vi "Fit.vi"(7 "Type X":T1(ring), 8 "error in (no error)":errorcluster caption="entrée d'erreur (pas d'erreur)", 9 "y":string[][](array[string]), 10 "X":string[][](array[string]), 11 "GaussianRandomProjection.lvclass":refnum<class "GaussianRandomProjection.lvclass">) -> (0 "error out":errorcluster caption="sortie d'erreur", 2 "String Data":string, 3 "GaussianRandomProjection.lvclass":refnum<class "GaussianRandomProjection.lvclass">)   [LabVIEW 2020, in "GaussianRandomProjection.lvclass"]
doc: "Generate a sparse random projection matrix\n\nReturns : \n\n- String : OK"
uses:
  GaussianRandomProjection.lvclass
  GaussianRandomProjection.lvclass/GaussianRandomProjection.ctl
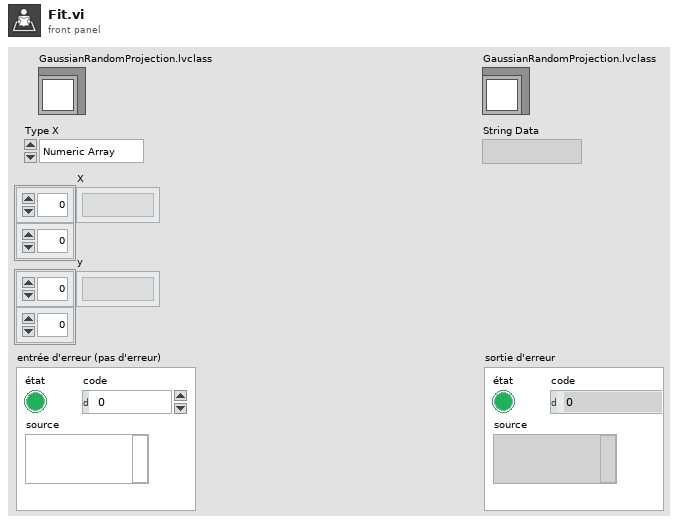
[diagram p1: front panel]
types:
  T1 = enum16{"Numeric Array", "String Array", "Sparse"}
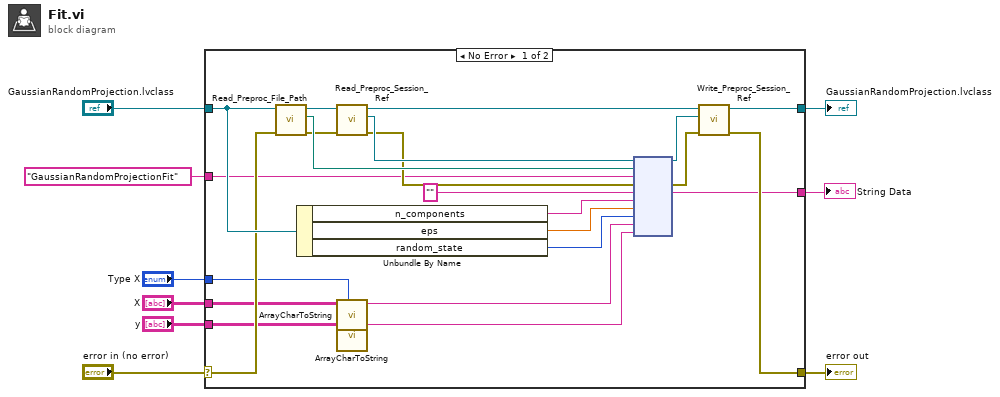
[diagram p0: block diagram]
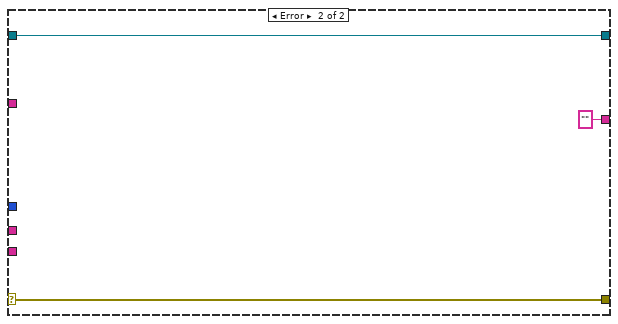
[diagram p2: hidden frame]
diagram:
  n1 = case shown="No Error" "error in (no error)" {
    selector: "error in (no error)" -> [w21 w35]
    tunnel: [w20 w35] -> w8
    tunnel: [w22 w34] -> w6
    tunnel: "GaussianRandomProjection.lvclass" -> [w23 w34]
    tunnel: "GaussianRandomProjectionFit" ("Fonction") -> [w19 _]
    tunnel: [w18 ""] -> w4
    tunnel: "X" -> [w14 _]
    tunnel: "y" -> [w13 _]
    tunnel: "Type X" -> [w12 _]
    frame No Error {
      n2 = call-dynamic "Read_Preproc_File_Path.vi"("error in (no error)"=w21, "Python in"=w23) -> ("error out"=w27:errorcluster, "File_Path"=w30:path, "Python out"=w32:refnum<class "GaussianRandomProjection.lvclass">)  [unwired: 7 in]
      n3 = Unbundle By Name(w23) -> ("n_components"=w17:string, "eps"=w16:dbl, "random_state"=w15:i32)
      n4 = call-dynamic "Read_Preproc_Session_Ref.vi"("error in (no error)"=w27, "Python in"=w32) -> ("error out"=w28:errorcluster, "Session_ref"=w29:refnum<k35>, "Python out"=w31:refnum<class "GaussianRandomProjection.lvclass">)  [unwired: 7 in]
      n5 = call "ArrayCharToString.vi"("Type"=w12, "TAB"=w14) -> ("Instruction"=w11:string)  [unwired: 9 in]
      n6 = call "ArrayCharToString.vi"("TAB"=w13) -> ("Instruction"=w10:string)  [unwired: 10 in]
      n7 = node(w29, w30, w19, w28, "", w17, w16, w15, w11, w10) -> (w24:refnum<k35>, w26:errorcluster, w18:string)  [unwired: 5 in, 2 out]
      n8 = call-dynamic "Write_Preproc_Session_Ref.vi"("error in (no error)"=w26, "Session_ref"=w24, "Python in"=w31) -> ("error out"=w20:errorcluster, "Python out"=w22:refnum<class "GaussianRandomProjection.lvclass">)  [unwired: 7 in]
    }
    frame Error {
    }
  }
  "error out" <- w8
  "GaussianRandomProjection.lvclass" <- w6
  "String Data" <- w4
